vi "Robot Main.vi"() -> ()   [LabVIEW 2013]
doc: "This VI imlements the framework and scheduler for your robotics program. It should not be necessary to modify the framework. You are expected to add your code to the VIs called from Robot Main, the ones located in the Team Code within the project."
uses:
  Robot Global Data.vi
panel:
  in  "Finish":bool
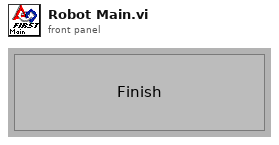
[diagram p1: front panel]
types:
  T1 = typedef "WPI_DriverStationMatch Info.ctl" = cluster{"Autonomous Elapsed Seconds":dbl, "TeleOp Elapsed Seconds":dbl, "Disabled Elapsed Seconds":dbl, "Visited Autonomous":bool, "Visited TeleOp":bool, "Visited Disabled":bool, "Autonomous Settings":cluster{"Autonomous Style":enum16{"Iterative", "Independent"}, "VI Refnum":refnum<vi>}}
  T2 = typedef "WPI_DriverStationDerivedRobotMode.ctl" = enum16{"Init", "Execute", "Stop"}
  T3 = typedef "WPI_DriverStationRobotMode2.ctl" = enum16{"Autonomous Disabled", "Autonomous Enabled", "Teleop Disabled", "Teleop Enabled", "Timeout", "Finish", "Test Disabled", "Test Enabled"}
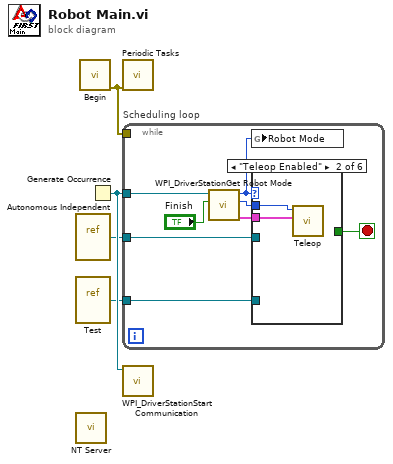
[diagram p0: block diagram]
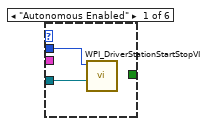
[diagram p2: hidden frame]
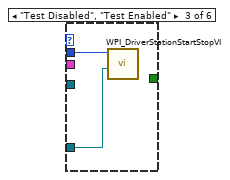
[diagram p3: hidden frame]
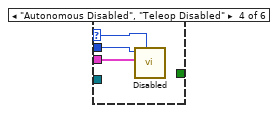
[diagram p4: hidden frame]
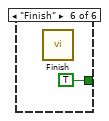
[diagram p6: hidden frame]
diagram:
  n1 = vi-ref "Autonomous Independent.vi"() -> (w3:refnum<vi>)
  n2 = vi-ref "Test.vi"() -> (w1:refnum<vi>)
  n3 = call <vilib>:"NT Server.vi"() -> ()  [unwired: 12 in]
  n4 = call "Begin.vi"() -> ("error out"=w2:errorcluster)  [unwired: 1 in, 10 out]
  n5 = Generate Occurrence() -> (w4:refnum<k4>)
  n6 = call "Periodic Tasks.vi"("error in"=w2) -> ()  [unwired: 1 in, 10 out]
  n7 = while "Scheduling loop" {
    tunnel: w4 -> [w11]
    tunnel: w2 -> [_]
    tunnel: w3 -> [w7]
    tunnel: w1 -> [w6]
    stop <- w8 stop-if-true
    n8 = call <vilib>:"WPI_DriverStationGet Robot Mode.vi"("Finish"="Finish", "DS Occurrence"=w11) -> ("Match Info out"=w9:T1, "Call Context"=w12:T2, "Robot Mode"=w5:T3)  [unwired: 7 out]
    n9 = global write "Robot Global Data.vi" "Robot Mode"(w5) -> ()
    n10 = case shown="\"Teleop Enabled\"" w5 {
      selector: w5 -> [_ _ _ w19 _ _]
      tunnel: w12 -> [w14 w16 w18 w21 _ _]
      tunnel: w9 -> [_ w15 _ w20 _ _]
      tunnel: [_ _ _ _ _ TRUE] -> w8
      tunnel: w7 -> [w13 _ _ _ _ _]
      tunnel: w6 -> [_ _ w17 _ _ _]
      frame "Autonomous Enabled" {
        n11 = call <vilib>:"WPI_DriverStationStartStopVI.vi"("VI in"=w13, "Call Context"=w14) -> ()  [unwired: 10 in]
      }
      frame "Teleop Enabled" {
        n12 = call "Teleop.vi"("Match Info"=w15, "Call Context"=w16) -> ()  [unwired: 1 in, 9 out]
      }
      frame "Test Disabled", "Test Enabled" {
        n13 = call <vilib>:"WPI_DriverStationStartStopVI.vi"("VI in"=w17, "Call Context"=w18) -> ()  [unwired: 10 in]
      }
      frame "Autonomous Disabled", "Teleop Disabled" {
        n14 = call "Disabled.vi"("Robot Mode"=w19, "Match Info"=w20, "Call Context"=w21) -> ()  [unwired: 1 in, 8 out]
      }
      frame "Timeout" {
      }
      frame "Finish" {
        n15 = call "Finish.vi"() -> ()  [unwired: 1 in, 7 out]
      }
    }
  }
  n16 = call <vilib>:"WPI_DriverStationStart Communication.vi"("occurrence"=w4) -> ()  [unwired: 11 out]
